vi "T1_KeyToValue.vi"(4 "Key":u64[](array[numeric]), 5 "String":string) -> (1 "Value":u64[](array[numeric]))   [LabVIEW 2022 SP3]
panel:
  out "Source > Dest":T1(c390)
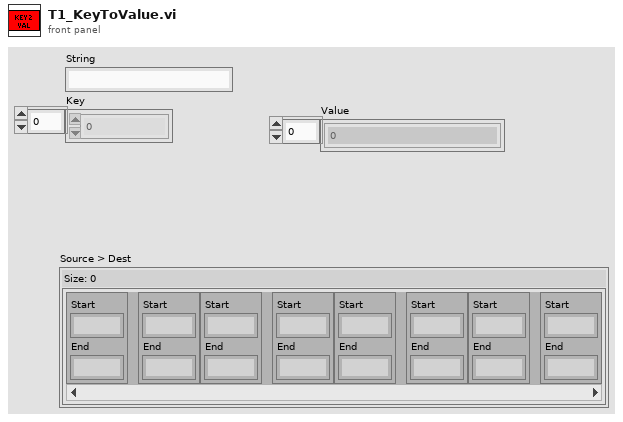
[diagram p1: front panel]
types:
  T1 = map{cluster{"Start":u64, "End":u64}, cluster{"Start":u64, "End":u64}}
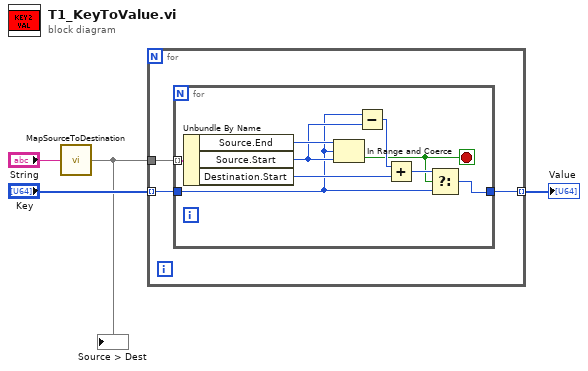
[diagram p0: block diagram]
diagram:
  n1 = call "MapSourceToDestination.vi"("String"="String") -> ("Source > Dest"=w2:T1)  [unwired: 6 in]
  "Source > Dest" <- w2
  n2 = for {
    tunnel: "Key" -> [w7] mode=indexing
    tunnel: w2 -> [w6]
    tunnel: [w5] -> w1 mode=indexing
    n3 = for {
      tunnel: w6 -> [w15] mode=indexing
      tunnel: w7 -> [w9]
      tunnel: [w8] -> w5
      stop <- w10 stop-if-true
      n4 = Unbundle By Name(w15) -> ("Source.End"=w16:u64, "Source.Start"=w14:u64, "Destination.Start"=w12:u64)
      n5 = In Range and Coerce(upper limit=w16, x=w9, lower limit=w14) -> (In Range?=w10:bool)  [unwired: 1 out]
      n6 = Subtract(x=w9, y=w14) -> (x-y=w13:u64)
      n7 = Add(x=w13, y=w12) -> (x+y=w11:u64)
      n8 = Select(t=w11, s=w10, f=w9) -> (s? t:f=w8:u64)
    }
  }
  "Value" <- w1
